vi "Simple Button Lamp Example.vi"() -> ()   [LabVIEW 2018]
uses:
  Lamp/Lamp.lvclass
  C:/GitClones/LGP5-Resources/LVOOP/Dependency-Inversion Principle/DIP/classes/Switchable Device/Switchable Device.lvclass
  Button/Button.lvclass
  Button/Button.lvclass/Button.ctl
  Switchable Device/Switchable Device.lvclass/Switchable Device.ctl
  Button/Set Button Pressed.vi
  Switchable Device/Get Is Turned ON.vi
  Switchable Device/Switchable Device.lvclass
panel:
  out "Lamp":bool
  in  "Button":bool
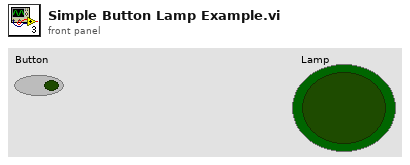
[diagram p1: front panel]
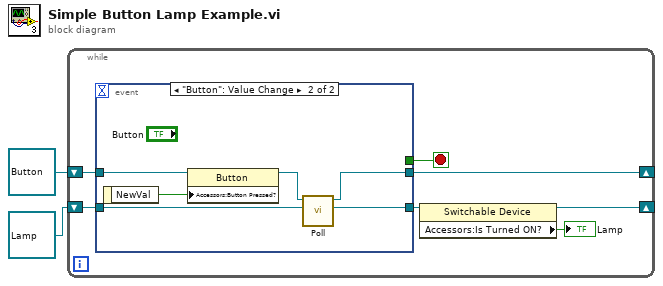
[diagram p0: block diagram]
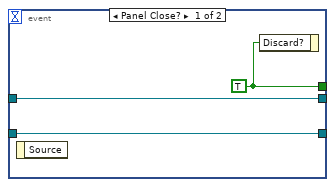
[diagram p2: hidden frame]
diagram:
  n1 = while {
    shift-right: [w6] -> _
    shift-left: refnum<class "Button.lvclass"> refnum ("Button in") -> [w8]
    shift-right: [w4] -> _
    shift-left: refnum<class "Lamp.lvclass"> refnum ("Lamp.lvclass") -> [w7]
    stop <- w9 stop-if-true
    n2 = event shown="[1] \"Button\": Value Change" {
      selector: _ -> [_ _]
      dyn-events: _ -> [_ _]
      timeout: _ -> [_ _]
      tunnel: [w12 _] -> w9
      tunnel: w8 -> [w11 w18]
      tunnel: w7 -> [w10 w15]
      tunnel: [w11 w14] -> w6
      tunnel: [w10 w13] -> w5
      event Panel Close? {
        w12 = TRUE ("Discard?")
        n3 = event-data() -> ()  [unwired: 1 in, 1 out]
        n4 = event-data("Discard?"=w12) -> ()  [unwired: 1 in, 1 out]
      }
      event "Button": Value Change {
        n5 = event-data() -> ("NewVal"=w16:bool)  [unwired: 1 in]
        n6 = property class="Button"(reference=w18, "Accessors:Button Pressed?"=w16) -> (reference out=w17:refnum<class "Button.lvclass">)  [unwired: 1 in, 1 out]
        n7 = call-dynamic "Poll.vi"("Switchable Device in"=w15, "Button in"=w17) -> ("Switchable Device out"=w13:refnum<class "Switchable Device.lvclass">, "Button out"=w14:refnum<class "Button.lvclass">)  [unwired: 7 in, 1 out]
      }
    }
    n8 = property class="Switchable Device"(reference=w5) -> (reference out=w4:refnum<class "Switchable Device.lvclass">, "Accessors:Is Turned ON?"=→"Lamp":bool)  [unwired: 1 in, 1 out]
  }
